vi "Checkers P2 Turn Drawer.vi"() -> (3 "new picture":picture)   [LabVIEW 2014]
uses:
  Game Info Global Variable.vi
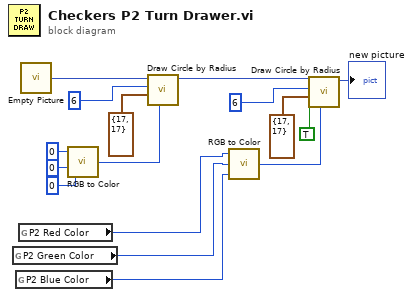
[diagram p0: block diagram]
diagram:
  n1 = global read "Game Info Global Variable.vi" "P2 Green Color"() -> (w2:i32)
  n2 = global read "Game Info Global Variable.vi" "P2 Blue Color"() -> (w3:i32)
  n3 = global read "Game Info Global Variable.vi" "P2 Red Color"() -> (w1:i32)
  n4 = call "Empty Picture"() -> ("empty picture"=w13:picture)
  n5 = call <vilib>:"RGB to Color.vi"("B"=u8 0, "G"=u8 0, "R"=u8 0) -> ("Color"=w16:u32)
  n6 = call <vilib>:"Draw Circle by Radius.vi"("color(black)"=w16, "pixel center"=cluster{"horizontal":i16, "vertical":i16} {"horizontal"=17, "vertical"=17}, "radius"=i16 6, "picture"=w13) -> ("new picture"=w6:picture)  [unwired: 7 in]
  n7 = call <vilib>:"RGB to Color.vi"("B"=w3, "G"=w2, "R"=w1) -> ("Color"=w7:u32)
  n8 = call <vilib>:"Draw Circle by Radius.vi"("color(black)"=w7, "fill?(F)"=TRUE, "pixel center"=cluster{"horizontal":i16, "vertical":i16} {"horizontal"=17, "vertical"=17}, "radius"=i16 6, "picture"=w6) -> ("new picture"=→"new picture":picture)  [unwired: 6 in]
